vi "Error Code Dialog.vi"(8 "error in":errorcluster) -> (0 "error out":errorcluster, 1 "Cancel Out":bool, 2 "Error Name":string)   [LabVIEW 2020, in "ConstantErrorsMaker.lvlib"]
uses:
  ConstantErrorsMaker.lvlib
  MulticolumListbox.ctl
  Continue.ctl
panel:
  in  "Project Ref":refnum<vi>
  in  "Main App Inst Ref":refnum<vi>
  in  "Library Ref":refnum<vi>
  in  "Error Description":string
  in  "Current Error VIs Values":T1
  in  "Error Name (do not add --error.vi)":string
  in  "Continue":T2
  in  "Cancel":bool
  in  "Error Code":i32
  # "These are the benefits of having Error Constant VIs\n\n1. Centralized Error Management:\n   - Single Point of Editing: by storing error codes and descriptions in constants, you can modify them in one place, ensuring consistency across the entire application. This streamlines maintenance and avoids potential errors due to inconsistencies.\n   - Enhanced Organization: Grouping error-related information in constants improves code readability and understanding. It also makes it easier to quickly locate and update error-related logic.\n\n2. Improved Code Readability:\n   - Clearer Meaning: Instead of using raw error codes directly in code, constants provide meaningful names for errors, making code more self-explanatory and easier for others to comprehend.\n   - Reduced Redundancy: Constants eliminate the need to repeatedly define error codes and descriptions throughout the code, reducing redundancy and improving code maintainability.\n\n3. Error Tracking and Debugging:\n   - Identifying Error Sources: By using constant VIs, you can easily track where specific errors are being generated within the application. This aids in debugging and pinpointing the root causes of issues.\n   - Debugging Efficiency: Constants make it easier to search for error-related code and analyze error handling logic, facilitating debugging and problem resolution.\n\n4. Flexibility for Customization:\n   - Adaptability: If error codes or descriptions need to change, you can easily update them in the constant VIs without having to modify code in multiple locations. This allows for quick adjustments and customization as needed.\n\nRanges of Custom Error Codes defined by NI:\n     –8999  through –8000\n       5000  through   9999\n  500,000  through 599,999"
  # "TIP: Doble click to open --error.vi Block Diagram"
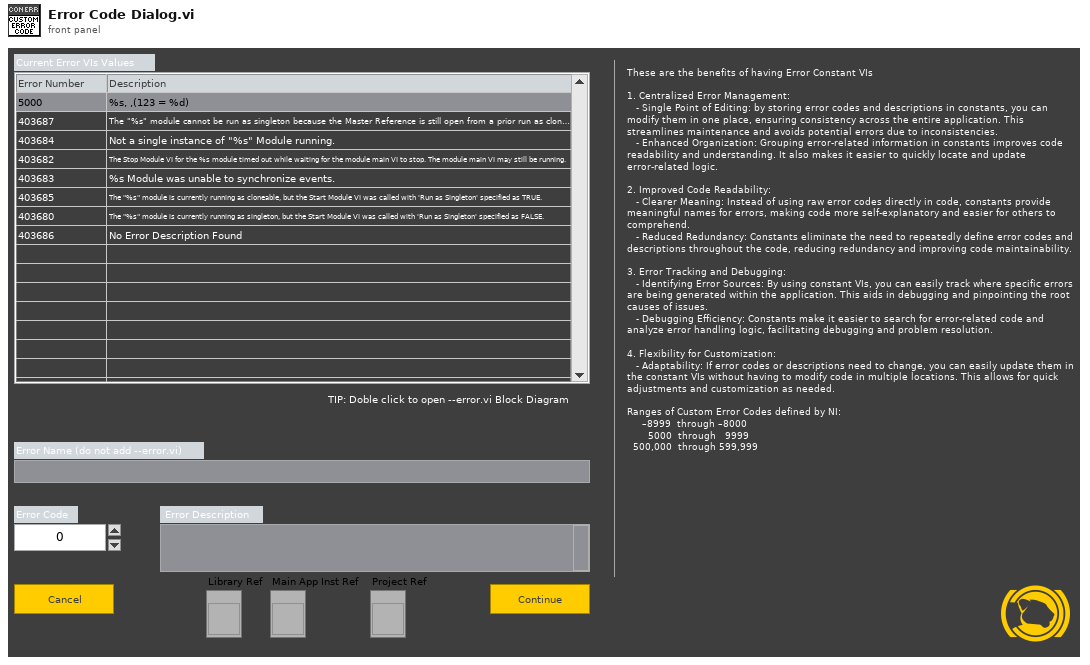
[diagram p1: front panel]
types:
  T1 = typedef "ConstantErrorsMaker.lvlib/MulticolumListbox.ctl" = i32
  T2 = typedef "ConstantErrorsMaker.lvlib/Continue.ctl" = bool
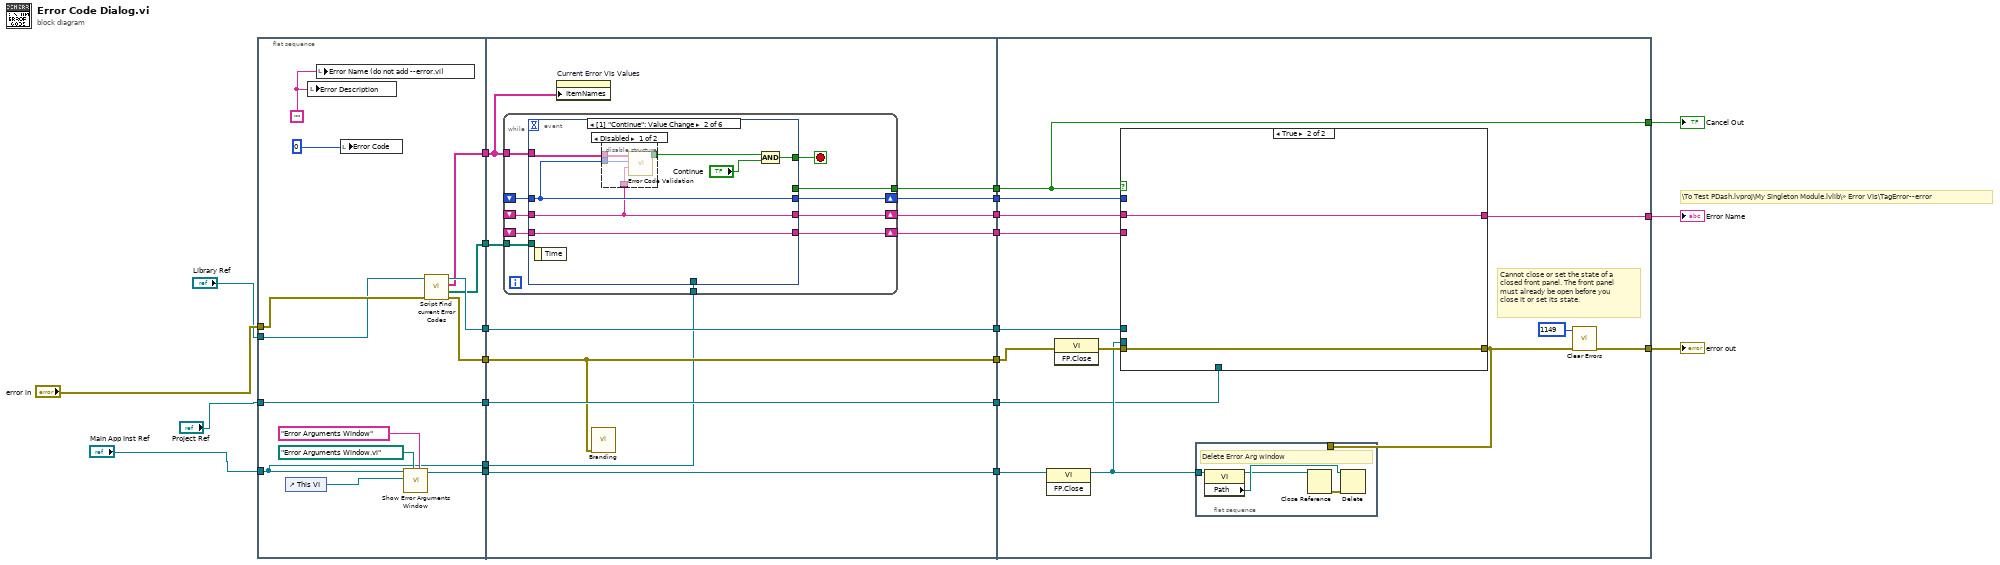
[diagram p0: block diagram]
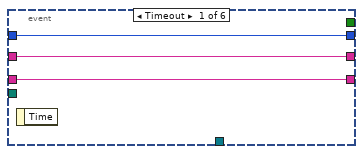
[diagram p2: hidden frame]
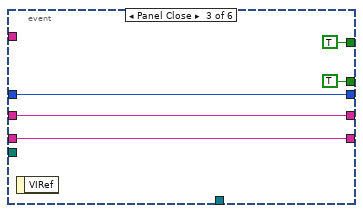
[diagram p4: hidden frame]
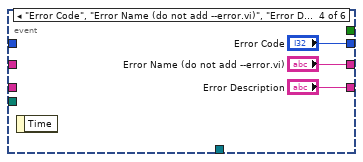
[diagram p5: hidden frame]
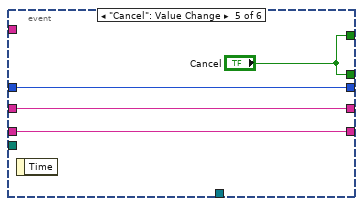
[diagram p6: hidden frame]
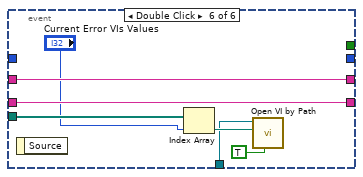
[diagram p7: hidden frame]
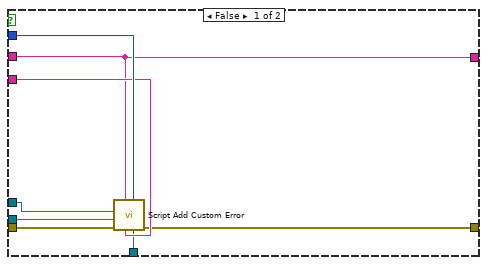
[diagram p8: hidden frame]
diagram:
  # "\\To Test PDash.lvproj\\My Singleton Module.lvlib\\» Error VIs\\TagError--error"
  n1 = flat-sequence {
    tunnel: "Library Ref" -> [w33]
    tunnel: "error in" -> [w36]
    tunnel: [w35] -> w22
    tunnel: [w32] -> w15
    tunnel: [w31] -> w14
    tunnel: [w29] -> w12
    tunnel: "Main App Inst Ref" -> [w23]
    tunnel: [w25] -> w9
    tunnel: "Project Ref" -> [w25]
    tunnel: [w24] -> w5
    tunnel: [w23] -> w4
    tunnel: w22 -> [w41]
    tunnel: [w41] -> w21
    tunnel: [w43] -> w19
    tunnel: [w47] -> w18
    tunnel: [w46] -> w17
    tunnel: [w45] -> w16
    tunnel: w15 -> [w45]
    tunnel: w14 -> [w40]
    tunnel: [w38] -> w13
    tunnel: w12 -> [w38]
    tunnel: [w44] -> w11
    tunnel: [w42] -> w10
    tunnel: w9 -> [w42]
    tunnel: w5 -> [w39]
    tunnel: w4 -> [w37]
    tunnel: [w105] -> w6
    tunnel: w21 -> [w102]
    tunnel: w19 -> [w92]
    tunnel: w18 -> [w101]
    tunnel: w17 -> [w100]
    tunnel: w16 -> [w99]
    tunnel: w13 -> [w97]
    tunnel: w11 -> [w95]
    tunnel: w10 -> [w94]
    tunnel: [w93] -> w8
    tunnel: [w92] -> w7
    frame #0 {
      w26 = "" ("Error Message")
      n2 = control-ref of="This VI"() -> (w30:refnum<vi>)
      n3 = local write "Error Description"(w26) -> ()
      n4 = local write "Error Name (do not add --error.vi)"(w26) -> ()
      n5 = local write "Error Code"(0 ("Error Code")) -> ()
      n6 = call "Show Error Arguments Window.vi"("Title"="Error Arguments Window", "Path"=path "Error Arguments Window.vi", "Calling VI Ref"=w30, "App Instance"=w23) -> ("Error Arguments Window Ref"=w29:refnum<vi>)  [unwired: 6 in, 1 out]
      n7 = call "Script Find current Error Codes.vi"("error in"=w36, "Library in"=w33) -> ("error out"=w35:errorcluster, "All Error VIS"=w24:path[], "Error and Descriptions Table"=w31:string[][], "Library out"=w32:refnum<vi>)  [unwired: 6 in]
    }
    frame #1 {
      n8 = while {
        shift-right: [w57] -> w46
        shift-left: _ -> [w56]
        shift-right: [w55] -> w47
        shift-left: _ -> [w54]
        tunnel: [w53] -> w43
        tunnel: w40 -> [w52]
        shift-right: [w51] -> w44
        shift-left: _ -> [w50]
        tunnel: w39 -> [w49]
        tunnel: w37 -> [w48]
        stop <- w58 stop-if-true
        n9 = event shown="[1] \"Continue\": Value Change" {
          selector: _ -> [_ _ _ _ _ _]
          dyn-events: _ -> [_ _ _ _ _ _]
          timeout: _ -> [_ _ _ _ _ _]
          tunnel: [_ w67 TRUE ("Cancel") _ "Cancel" _] -> w58
          tunnel: [w61 w68 w73 "Error Code" w83 _] -> w57
          tunnel: w56 -> [w61 w68 w73 _ w83 _]
          tunnel: [w60 w62 w77 "Error Name (do not add --error.vi)" w84 w91] -> w55
          tunnel: w54 -> [w60 w62 w77 _ w84 w91]
          tunnel: [_ _ TRUE ("Cancel") _ "Cancel" _] -> w53
          tunnel: w52 -> [_ w64 _ _ _ _]
          tunnel: [w59 w63 w74 "Error Description" w81 w90] -> w51
          tunnel: w50 -> [w59 w63 w74 _ w81 w90]
          tunnel: w49 -> [_ _ _ _ _ w89]
          tunnel: w48 -> [_ _ _ _ _ w86]
          event Timeout {
            n10 = event-data() -> ()  [unwired: 1 in, 1 out]
          }
          event Value Change {
            n11 = event-data() -> ()  [unwired: 1 in, 1 out]
            n12 = disable-structure shown="Disabled" {
              disable-tunnel: w68 -> [w72 _]
              disable-tunnel: [w71 _] -> w65
              disable-tunnel: w64 -> [w70 _]
              disable-tunnel: w62 -> [w69 _]
              frame Disabled {
                n13 = call "Error Code Validation.vi"("Error Name"=w69, "New Error Code"=w72, "Error Codes and Descriptions"=w70) -> ("Continue"=w71:bool)  [unwired: 8 in]
              }
              frame Enabled {
              }
            }
            n14 = And(x=w65, y="Continue") -> (x .and. y?=w67:T2)
          }
          event Panel Close {
            n15 = event-data() -> ()  [unwired: 1 in, 1 out]
          }
          event "Error Code", "Error Name (do not add --error.vi)", "Error Description": Value Change {
            n16 = event-data() -> ()  [unwired: 1 in, 1 out]
          }
          event "Cancel": Value Change {
            n17 = event-data() -> ()  [unwired: 1 in, 1 out]
          }
          event Double Click {
            n18 = event-data() -> ()  [unwired: 1 in, 1 out]
            n19 = Index Array(array=w89, index="Current Error VIs Values") -> (element=w87:path)
            n20 = call "Open VI by Path.vi"("Block Diagram?"=TRUE, "VI Path"=w87, "Application in"=w86) -> ()  [unwired: 8 in, 1 out]
          }
        }
      }
      n21 = property on="Current Error VIs Values" class="MCListbox (strict)"("ItemNames"=w40) -> ()  [unwired: 2 in, 2 out]
      n22 = call "Branding.vi"("error in"=w41) -> ()  [unwired: 11 in]
    }
    frame #2 {
      # "Cannot close or set the state of a closed front panel. The front panel must already be open before you close it or set its state."
      n23 = invoke class="VI" method="FP.Close"(reference=w97) -> (reference out=w96:refnum<vi>)  [unwired: 2 in, 2 out]
      n24 = invoke class="VI" method="FP.Close"(error in=w102) -> (error out=w104:errorcluster)  [unwired: 2 in, 2 out]
      n25 = case shown="True" w92 {
        tunnel: [w110 w119] -> w103
        tunnel: w104 -> [w117 w119]
        tunnel: w101 -> [w111 w118]
        tunnel: w100 -> [w116 _]
        tunnel: w99 -> [w115 _]
        tunnel: w96 -> [w114 _]
        tunnel: w95 -> [w113 _]
        tunnel: w94 -> [w112 _]
        tunnel: [w111 w118] -> w93
        frame False {
          n26 = call "Script Add Custom Error.vi"("Project Reference"=w112, "Error Code"=w116, "Error Description"=w113, "Error Name"=w111, "error in"=w117, "Error Arguments Window Ref"=w114, "DQMH Lib Ref"=w115) -> ("error out"=w110:errorcluster)  [unwired: 4 in]
        }
        frame True {
        }
      }
      n27 = flat-sequence {
        tunnel: w96 -> [w108]
        tunnel: w103 -> [_]
        frame #0 {
          # "Delete Error Arg window"
          n28 = property class="VI"(reference=w108) -> (reference out=w106:refnum<vi>, "Path"=w107:path)  [unwired: 1 in, 1 out]
          n29 = Close Reference(reference=w106) -> (error out=w109:errorcluster)  [unwired: 1 in]
          n30 = Delete(path (use dialog)=w107, error in=w109) -> ()  [unwired: 3 in, 3 out]
        }
      }
      n31 = call <vilib>:"Clear Errors.vi"("error in (no error)"=w103, "specific error code to clear (0: all)"=1149) -> ("error out"=w105:errorcluster)  [unwired: 4 in, 1 out]
    }
  }
  "error out" <- w6
  "Error Name" <- w8
  "Cancel Out" <- w7
